vi "Side VErtical Minimum.vi"(0 "Image":T8, 1 "Calibrated Image":T8, 3 "Ellipse Center":cluster{"Center X":dbl, "Center Y":dbl}, 4 "Search Direction ROI Ref":u32(ring) items=["Left to Right", "Right to Left", "Top to Bottom", "Bottom to Top"], 5 "Edge Options ROI Ref":T1={"Edge Polarity"=0, "Kernel Size"=3, "Width"=3, "Minimum Edge Strength"=10.0, "Interpolation Type"=enum."Bilinear Fixed", "Data Processing Method"=enum."Average"} {"Edge Polarity" items=["All Edges", "Rising Edges", "Falling Edges"]; "Minimum Edge Strength" format="%.2f"; "Width" step=2; "Kernel Size" step=2}, 7 "error in (no error)":errorcluster, 9 "ROI 1 Edge Strength":i32, 10 "Line Options ROI Ref":T5={"Number of Lines"=1, "Type"=enum."Best Edge Projection", "Min. Score"=10.0, "Max. Score"=1000.0, "Orientation"=0.0, "Angle Range"=10.0, "Angle Tolerance"=1.0, "Step Size"=3, "Min. SNR (db)"=0.0, "Min. Points (%)"=25.0, "Hough Iterations"=5} {"Min. Points (%)" min=0.0 max=100.0; "Min. SNR (db)" min=0.0; "Max. Score" min=0.0 max=1024.0; "Min. Score" min=0.0 max=1024.0 step=1.0}, 11 "Edge Options ROI 1":T1={"Edge Polarity"=0, "Kernel Size"=3, "Width"=3, "Minimum Edge Strength"=50.0, "Interpolation Type"=enum."Zero Order", "Data Processing Method"=enum."Average"} {"Edge Polarity" items=["All Edges", "Rising Edges", "Falling Edges"]; "Minimum Edge Strength" format="%.2f"; "Width" step=2; "Kernel Size" step=2}, 12 "Ref ROI after Transformation SV":T7 {"Contours"."Type" items=["No Selection", "Point", "Line", "Rectangle", "Oval", "Polygon", "Free", "Annulus", "Unused2", "Unused3", "Broken Line", "Free Hand Line", "Rotated Rectangle"]}, 13 "Meas ROI 1 Before Transformation":T4 {"Contours"."Type" items=["No Selection", "Point", "Line", "Rectangle", "Oval", "Polygon", "Freehand Region", "Annulus", "Unused2", "Unused3", "Broken Line", "Freehand Line", "Rotated Rectangle"]}, 14 "ROI 1Step Size":u32, 15 "Overlay Boolean Cluster":T3={"Overlay ROI"=TRUE, "Overlay Edge/ Points"=TRUE, "Overlay Rake Lines"=TRUE}) -> (18 "Edge Coordinates":cluster{"X":sgl, "Y":sgl}[](array[cluster]) {"Y" format="%.2f"; "X" format="%.2f"}, 20 "Numeric":sgl, 27 "error out":errorcluster)   [LabVIEW 2019, in "Algorithm.lvclass"]
uses:
  FrameworkOverrides/Algorithm.lvclass
  <vilib>/vision/NI_Vision_Development_Module.lvlib
  <vilib>/vision/Image Controls.llb/IMAQ Image.ctl
  <vilib>/vision/Measure.llb/Edge Polarity.ctl
  <vilib>/vision/Measure.llb/Edge Options.ctl
  <vilib>/vision/Measure.llb/Straight Edge Process.ctl
  <vilib>/vision/Measure.llb/Straight Edge Options.ctl
panel:
  out "Array":sgl[](array[numeric])
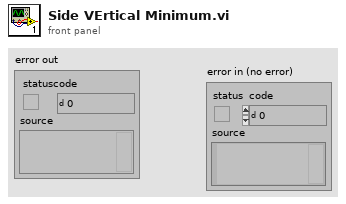
[diagram p1: front panel]
types:
  T1 = typedef "Edge Options.ctl" = cluster{"Edge Polarity":T2, "Kernel Size":u32, "Width":u32, "Minimum Edge Strength":sgl, "Interpolation Type":enum32{"Zero Order", "Bilinear", "Quadratic", "Cubic", "Bilinear Fixed"}, "Data Processing Method":enum32{"Average", "Median"}}
  T2 = typedef "Edge Polarity.ctl" = u32
  T3 = cluster{"Overlay ROI":bool, "Overlay Edge/ Points":bool, "Overlay Rake Lines":bool}
  T4 = typedef "ROI Descriptor" = cluster{"Global Rectangle":i32[], "Contours":cluster{"ID":enum32{"External", "Internal"}, "Type":u32, "Coordinates":i32[]}[]}
  T5 = typedef "Straight Edge Options.ctl" = cluster{"Number of Lines":i32, "Type":T6, "Min. Score":dbl, "Max. Score":dbl, "Orientation":dbl, "Angle Range":dbl, "Angle Tolerance":dbl, "Step Size":u32, "Min. SNR (db)":dbl, "Min. Points (%)":dbl, "Hough Iterations":i32}
  T6 = typedef "Straight Edge Process.ctl" = enum32{"First Edge Rake", "Best Edge Rake", "Hough Edge Rake", "First Edge Projection", "Best Edge Projection"}
  T7 = cluster{"Global Rectangle":i32[], "Contours":cluster{"ID":enum32{"External", "Internal"}, "Type":u32, "Coordinates":i32[]}[]}
  T8 = typedef "IMAQ Image.ctl" = refnum<image>
  T9 = typedef "IMAQ Rectangle" = cluster{"Left":i32, "Top":i32, "Right":i32, "Bottom":i32, "Rotation":dbl}
  T10 = cluster{"Contrast":i32, "Filter width":i32, "Steepness":i32, "Subsampling Ratio":u32, "Show Search Area":bool, "Show Search Lines":bool, "Show Edges Found":bool, "Show Result":bool}
  T11 = cluster{"Point1 (Pixels)":cluster{"X":sgl, "Y":sgl}, "Point2 (Pixels)":cluster{"X":sgl, "Y":sgl}, "Point1 (Real-World)":cluster{"X":sgl, "Y":sgl}, "Point2 (Real-World)":cluster{"X":sgl, "Y":sgl}, "Angle (Pixel)":dbl, "Angle (Real-World)":dbl, "Score":dbl, "Straightness":dbl, "Average SNR (db)":dbl, "Calibration Valid":bool}[]
  T12 = cluster{"Left":dbl, "Top":dbl, "Right":dbl, "Bottom":dbl, "Angle":dbl}
  T13 = typedef "Search Line.ctl" = cluster{"Start Point":cluster{"X":sgl, "Y":sgl}, "End Point":cluster{"X":sgl, "Y":sgl}, "Edge Info":T14[], "Edge Map":dbl[], "Calibration Valid":bool}
  T14 = typedef "Edge New.ctl" = cluster{"Location (Pixel)":cluster{"X":sgl, "Y":sgl}, "Location (Real-World)":cluster{"X":sgl, "Y":sgl}, "Distance (Pixel)":dbl, "Distance (Real-World)":dbl, "Strength":dbl, "Noise":dbl, "Rising?":bool}
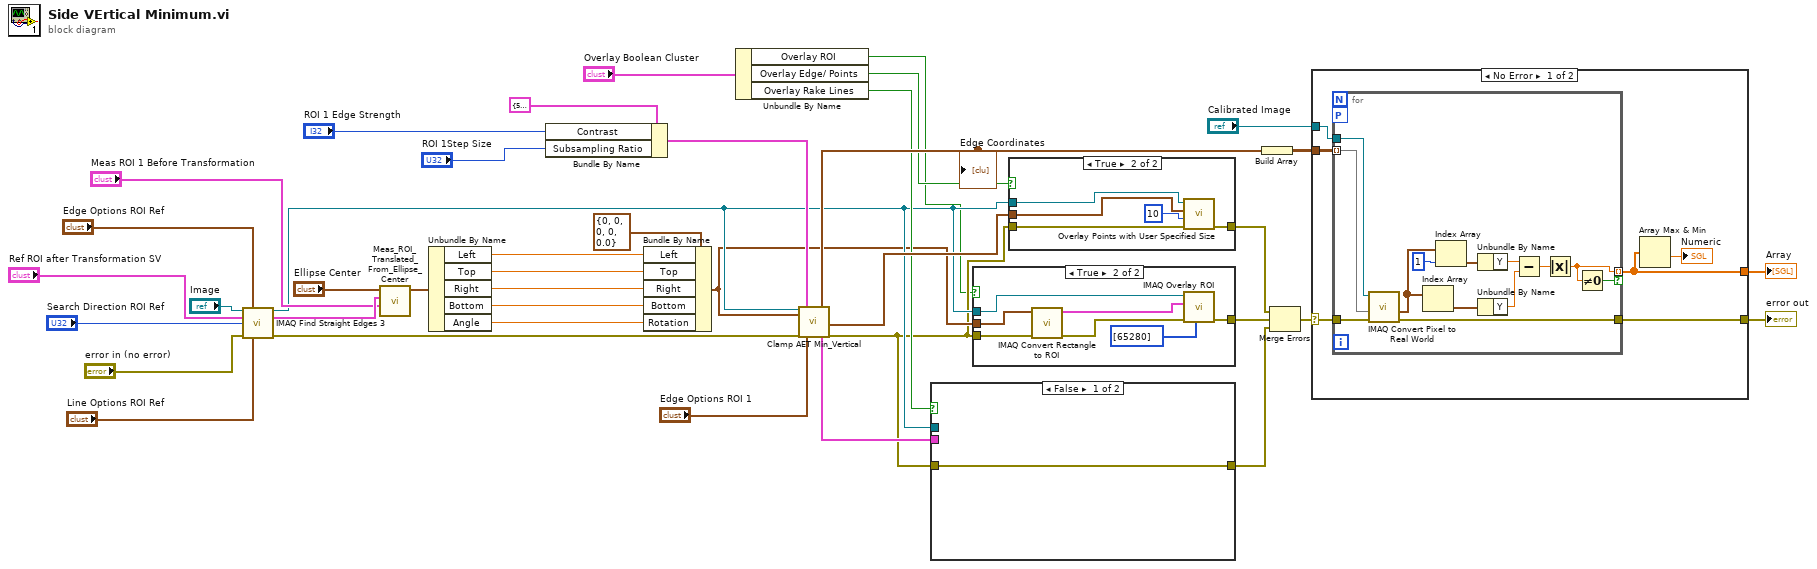
[diagram p0: block diagram]
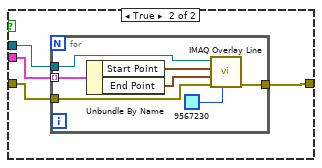
[diagram p2: hidden frame]
diagram:
  n1 = call "IMAQ Find Straight Edges 3"("Image"="Image", "Edge Options"="Edge Options ROI Ref", "ROI Descriptor"="Ref ROI after Transformation SV", "Search Direction"="Search Direction ROI Ref", "error in (no error)"="error in (no error)", "Line Options"="Line Options ROI Ref") -> ("Image (duplicate)"=w8:T8, "Straight Edges"=w30:T11, "error out"=w21:errorcluster)  [unwired: 5 in, 2 out]
  n2 = call "Meas_ROI_Translated_From_Ellipse_Center.vi"("ROI Descriptor"="Meas ROI 1 Before Transformation", "Straight Edges"=w30, "Ellipse Center"="Ellipse Center") -> ("Translated ROI"=w27:T12)  [unwired: 8 in]
  n3 = Unbundle By Name(w27) -> ("Left"=w26:dbl, "Top"=w25:dbl, "Right"=w24:dbl, "Bottom"=w23:dbl, "Angle"=w22:dbl)
  n4 = Bundle By Name(cluster=T10 {"Contrast"=50, "Filter width"=4, "Steepness"=2, "Subsampling Ratio"=5, "Show Search Area"=FALSE, "Show Search Lines"=FALSE, "Show Edges Found"=FALSE, "Show Result"=FALSE} ("Settings"), "Contrast"="ROI 1 Edge Strength", "Subsampling Ratio"="ROI 1Step Size") -> (w20:T10)
  n5 = Bundle By Name(cluster=T9 {"Left"=0, "Top"=0, "Right"=0, "Bottom"=0, "Rotation"=0.0} ("Rectangle"), "Left"=w26, "Top"=w25, "Right"=w24, "Bottom"=w23, "Rotation"=w22) -> (w7:T9)
  n6 = Unbundle By Name("Overlay Boolean Cluster") -> ("Overlay ROI"=w2:bool, "Overlay Edge/ Points"=w12:bool, "Overlay Rake Lines"=w11:bool)
  n7 = call "Clamp AET Min_Vertical.vi"("Image"=w8, "Rectangle"=w7, "error in (no error)"=w21, "Settings"=w20, "Edge Options"="Edge Options ROI 1") -> ("Edge Coordinates"=w17:cluster{"X":sgl, "Y":sgl}[], "Search Lines"=w10:T13[], "First and Last Edge Points"=w13:cluster{"X":sgl, "Y":sgl}[], "error out"=w5:errorcluster)  [unwired: 6 in, 5 out]
  "Edge Coordinates" <- w17
  n8 = case shown="False" w11 {
    tunnel: w10 -> [_ w45]
    tunnel: w8 -> [_ w44]
    tunnel: w5 -> [w41 w43]
    tunnel: [w41 w42] -> w4
    frame False {
    }
    frame True {
      n9 = for {
        tunnel: w45 -> [w52] mode=indexing
        tunnel: w44 -> [w48]
        tunnel: w43 -> [w47]
        tunnel: [w46] -> w42
        n10 = Unbundle By Name(w52) -> ("Start Point"=w51:cluster{"X":sgl, "Y":sgl}, "End Point"=w50:cluster{"X":sgl, "Y":sgl})
        n11 = call "IMAQ Overlay Line"("Color"=u32 9567230, "error in (no error)"=w47, "End Point"=w50, "Start Point"=w51, "Image"=w48) -> ("error out"=w46:errorcluster)  [unwired: 5 in, 1 out]
      }
    }
  }
  n12 = case shown="True" w2 {
    tunnel: w8 -> [_ w60]
    tunnel: w7 -> [_ w59]
    tunnel: [w53 w56] -> w6
    tunnel: w5 -> [w53 w55]
    frame False {
    }
    frame True {
      n13 = call "IMAQ Convert Rectangle to ROI"("error in (no error)"=w55, "Rectangle"=w59) -> ("error out"=w54:errorcluster, "ROI Descriptor"=w58:T4)  [unwired: 7 in]
      n14 = call "IMAQ Overlay ROI"("Colors (Green)"=u32[] [65280], "error in (no error)"=w54, "ROI Descriptor"=w58, "Image"=w60) -> ("error out"=w56:errorcluster)  [unwired: 6 in, 1 out]
    }
  }
  n15 = case shown="True" w12 {
    tunnel: w13 -> [_ w66]
    tunnel: w8 -> [_ w65]
    tunnel: [w61 w63] -> w9
    tunnel: w5 -> [w61 w62]
    frame False {
    }
    frame True {
      n16 = call "Overlay Points with User Specified Size.vi"("error in"=w62, "Point Diameter (5)"=u32 10, "Points"=w66, "Image In"=w65) -> ("error out"=w63:errorcluster)  [unwired: 6 in, 1 out]
    }
  }
  n17 = Build Array(w17) -> (w16:cluster{"X":sgl, "Y":sgl}[][])
  n18 = Merge Errors(w9, w6, w4) -> (w3:errorcluster)
  n19 = case shown="No Error" w3 {
    selector: w3 -> [w72 w86]
    tunnel: [w71 w86] -> w15
    tunnel: [w70 _] -> w19
    tunnel: "Calibrated Image" -> [w68 _]
    tunnel: w16 -> [w67 _]
    frame No Error {
      n20 = for {
        tunnel: w67 -> [w85] mode=indexing
        tunnel: w68 -> [w84]
        tunnel: [w79] -> w70 mode=indexing if=w80
        tunnel: w72 -> [w82]
        tunnel: [w81] -> w71
        workers-P: _ -> [_]
        n21 = call "IMAQ Convert Pixel to Real World"("error in (no error)"=w82, "Array of Pixel Coordinates"=w85, "Calibrated Image"=w84) -> ("error out"=w81:errorcluster, "Array of Real World Coordinates"=w83:cluster{"X":sgl, "Y":sgl}[])  [unwired: 3 in, 4 out]
        n22 = Index Array(array=w83) -> (element=w78:cluster{"X":sgl, "Y":sgl})  [unwired: 1 in]
        n23 = Index Array(array=w83, index=1) -> (element=w76:cluster{"X":sgl, "Y":sgl})
        n24 = Unbundle By Name(w76) -> ("Y"=w75:sgl)
        n25 = Unbundle By Name(w78) -> ("Y"=w77:sgl)
        n26 = Subtract(x=w75, y=w77) -> (x-y=w73:sgl)
        n27 = Absolute Value(x=w73) -> (abs(x)=w79:sgl)
        n28 = Not Equal To 0?(x=w79) -> (x != 0?=w80:bool)
      }
      n29 = Array Max & Min(array=w70) -> (min value=→"Numeric":sgl)  [unwired: 3 out]
    }
    frame Error {
    }
  }
  "error out" <- w15
  "Array" <- w19
